vi "qc4_rafik_psm_Aurduino.vi"() -> ()   [LabVIEW 2020]
uses:
  <instrlib>/CAEN PSM/CAEN PSM.lvlib
panel:
  out "millisecond timer value":u32
  in  "Parameter name":string
  in  "Board parameter? (F)":bool
  out "Parameter descriptor":T1
  out "VMon display":dbl[](array[numeric]) format="%.1f"
  out "Vset DISP":dbl
  out "loop count":i32
  out "IMon values (uA)":dbl[][](array[numeric])
  out "Req (cal Mohm)":dbl[][](array[numeric])
  out "VMon values (V)":dbl[][](array[numeric])
  in  "Voltage Max (0.0 V) 2":u16 max=9999
  in  "Enable (OFF)":bool
  in  "Vinital Value(V)":dbl
  in  "Req (Mohm)":dbl
  in  "Board Address":i8
  in  "Channel (0)":u8
  in  "CAEN N1470/1471 PORT":refnum<visa-resource-name>
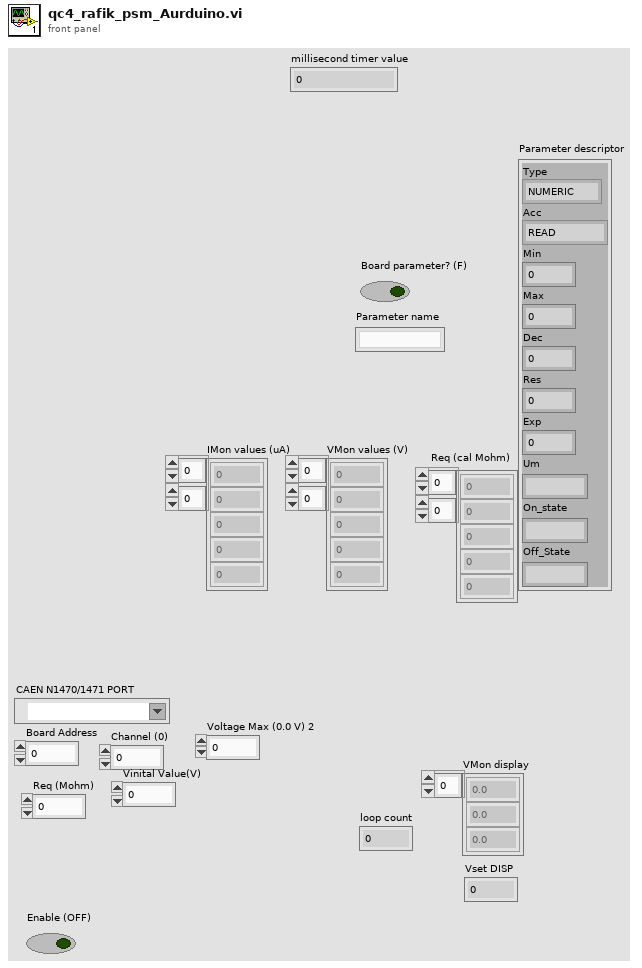
[diagram p1: front panel]
types:
  T1 = cluster{"Type":enum16{"NUMERIC", "ONOFF", "CHSTATUS", "BDSTATUS", "BINARY", "STRING", "ENUM"}, "Acc":enum16{"READ", "WRITE", "READ_WRITE"}, "Min":u32, "Max":u32, "Dec":u32, "Res":u32, "Exp":i32, "Um":string, "On_state":string, "Off_State":string}
  T2 = cluster{"Baud Rate":u32, "Parity":enum16{"None", "Odd", "Even", "Mark", "Space"}, "Data Bits":u16, "Stop Bits":u16, "Flow Control":u16}
  T3 = typedef "CAEN PSM.lvlib/BoardHandle.ctl" = cluster{"VISA resource name":refnum<visa-resource-name>, "Board address":i8, "NChannels":u8}
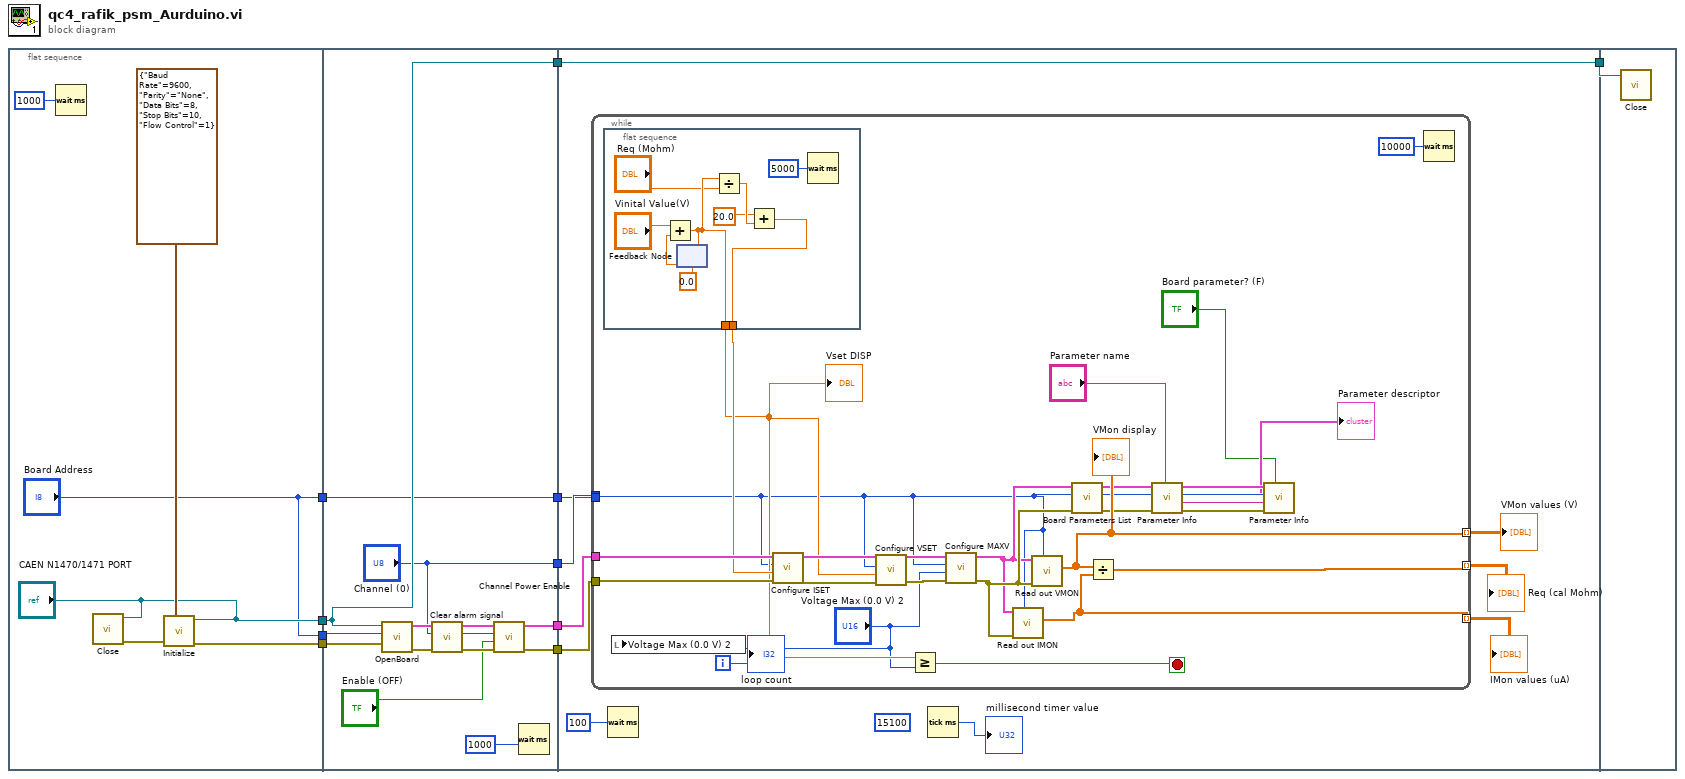
[diagram p0: block diagram]
diagram:
  n1 = flat-sequence {
    tunnel: [w13] -> w10
    tunnel: ["CAEN N1470/1471 PORT"] -> w9
    tunnel: ["Board Address"] -> w7
    tunnel: ["Board Address"] -> w5
    tunnel: w10 -> [w29]
    tunnel: w9 -> [w28]
    tunnel: [w28] -> w8
    tunnel: w7 -> [w27]
    tunnel: [w27] -> w6
    tunnel: w5 -> [w22]
    tunnel: [w21] -> w4
    tunnel: [w20] -> w3
    tunnel: ["Channel (0)"] -> w2
    tunnel: w8 -> [w34]
    tunnel: w6 -> [w32]
    tunnel: w4 -> [w37]
    tunnel: w3 -> [w38]
    tunnel: w2 -> [w39]
    tunnel: [w34] -> w1
    tunnel: w1 -> [w74]
    frame #0 {
      n2 = Wait (ms)(milliseconds to wait=u32 1000) -> ()  [unwired: 1 out]
      n3 = call <instrlib>:"Close.vi"("VISA resource name"="CAEN N1470/1471 PORT") -> ("error out"=w16:errorcluster)  [unwired: 10 in]
      n4 = call <instrlib>:"Initialize.vi"("Serial Configuration"=T2 {"Baud Rate"=9600, "Parity"=enum."None", "Data Bits"=8, "Stop Bits"=10, "Flow Control"=1}, "error in (no error)"=w16, "VISA resource name"="CAEN N1470/1471 PORT") -> ("error out"=w13:errorcluster)  [unwired: 7 in, 1 out]
    }
    frame #1 {
      n5 = call <instrlib>:"OpenBoard.vi"("error in (no error)"=w29, "Board Address"=w22, "VISA resource name"=w28) -> ("error out"=w25:errorcluster, "BoardHandle"=w26:T3)  [unwired: 7 in]
      n6 = call <instrlib>:"Clear alarm signal.vi"("error in (no error)"=w25, "BoardHandle"=w26) -> ("error out"=w24:errorcluster, "BoardHandle out"=w23:T3)  [unwired: 8 in]
      n7 = call <instrlib>:"Channel Power Enable.vi"("error in (no error)"=w24, "Enable (OFF)"="Enable (OFF)", "Channel (0)"="Channel (0)", "BoardHandle"=w23) -> ("error out"=w20:errorcluster, "BoardHandle out"=w21:T3)  [unwired: 6 in]
      n8 = Wait (ms)(milliseconds to wait=u32 1000) -> ()  [unwired: 1 out]
    }
    frame #2 {
      (unwired) u32 15100 ("millisecond timer value")
      n9 = while {
        tunnel: w39 -> [w44]
        tunnel: w38 -> [w60]
        tunnel: w37 -> [w59]
        tunnel: [w57] -> w36 mode=indexing
        tunnel: [w56] -> w33 mode=indexing
        tunnel: [w55] -> w35 mode=indexing
        tunnel: w32 -> [_]
        i -> [w52]
        stop <- w53 stop-if-true
        n10 = flat-sequence {
          tunnel: [w73] -> w58
          tunnel: [w72] -> w54
          frame #0 {
            n11 = feedback #1(0.0) -> (w70:dbl)
            n12 = Add(x="Vinital Value(V)", y=w70) -> (x+y=w72:dbl)
            n13 = feedback-in #1(w72) -> ()
            n14 = Divide(x=w72, y="Req (Mohm)") -> (x/y=w68:dbl)
            n15 = Add(x=20.0, y=w68) -> (x+y=w73:dbl)
            n16 = Wait (ms)(milliseconds to wait=u32 5000) -> ()  [unwired: 1 out]
          }
        }
        n17 = local write "Voltage Max (0.0 V) 2"("Voltage Max (0.0 V) 2") -> ()
        n18 = call <instrlib>:"Configure ISET.vi"("error in (no error)"=w60, "Current Limit (0.00 uA)"=w58, "Channel (0)"=w44, "BoardHandle"=w59) -> ("error out"=w62:errorcluster, "BoardHandle out"=w61:T3)  [unwired: 6 in]
        n19 = call <instrlib>:"Configure VSET.vi"("error in (no error)"=w62, "Voltage Level (0.0 V)"=w54, "Channel (0)"=w44, "BoardHandle"=w61) -> ("error out"=w64:errorcluster, "BoardHandle out"=w63:T3)  [unwired: 6 in]
        n20 = Greater Or Equal?(x=w54, y="Voltage Max (0.0 V) 2") -> (x >= y?=w53:bool)
        n21 = call <instrlib>:"Configure MAXV.vi"("error in (no error)"=w64, "Voltage Max (0.0 V)"="Voltage Max (0.0 V) 2", "Channel (0)"=w44, "BoardHandle"=w63) -> ("error out"=w50:errorcluster, "BoardHandle out"=w49:T3)  [unwired: 6 in]
        n22 = call <instrlib>:"Read out IMON.vi"("Channel"=w44, "error in (no error)"=w50, "BoardHandle"=w49) -> ("IMon values (uA)"=w55:dbl[])  [unwired: 5 in, 3 out]
        n23 = call <instrlib>:"Read out VMON.vi"("Channel"=w44, "error in (no error)"=w50, "BoardHandle"=w49) -> ("VMon values (V)"=w56:dbl[])  [unwired: 6 in, 2 out]
        "VMon display" <- w56
        n24 = call <instrlib>:"Board Parameters List.vi"("error in (no error)"=w50, "BoardHandle"=w49) -> ("error out"=w47:errorcluster, "BoardHandle out"=w48:T3)  [unwired: 6 in, 2 out]
        n25 = Divide(x=w56, y=w55) -> (x/y=w57:dbl[])
        n26 = call <instrlib>:"Parameter Info.vi"("error in (no error)"=w47, "Parameter name"="Parameter name", "Channel"=w44, "BoardHandle"=w48) -> ("error out"=w45:errorcluster, "BoardHandle out"=w46:T3)  [unwired: 5 in, 1 out]
        n27 = call <instrlib>:"Parameter Info.vi"("Board parameter? (F)"="Board parameter? (F)", "error in (no error)"=w45, "Parameter name"="Parameter name", "Channel"=w44, "BoardHandle"=w46) -> ("Parameter descriptor"=→"Parameter descriptor":T1)  [unwired: 4 in, 2 out]
        n28 = Wait (ms)(milliseconds to wait=u32 10000) -> ()  [unwired: 1 out]
        "loop count" <- w52
        "Vset DISP" <- w54
      }
      "VMon values (V)" <- w33
      "Req (cal Mohm)" <- w36
      "IMon values (uA)" <- w35
      n29 = Wait (ms)(milliseconds to wait=u32 100) -> ()  [unwired: 1 out]
      n30 = Tick Count (ms)() -> (millisecond timer value=→"millisecond timer value":u32)
    }
    frame #3 {
      n31 = call <instrlib>:"Close.vi"("VISA resource name"=w74) -> ()  [unwired: 10 in, 1 out]
    }
  }
